vi "ajouterdonneeuser.vi"(0 "Validation":bool, 1 "Nom":string, 2 "Fichier DB":string, 3 "Prénom":string, 4 "Code du poste":dbl) -> ()   [LabVIEW 2024]
uses:
  <vilib>/drjdpowell/SQLite Library/SQL Connection/Open (string).vi
  <vilib>/drjdpowell/SQLite Library/SQL Connection/Execute SQL (No results).vi
  <vilib>/drjdpowell/SQLite Library/SQL Connection/Connection.lvclass
  <vilib>/drjdpowell/SQLite Library/SQLite.lvlib
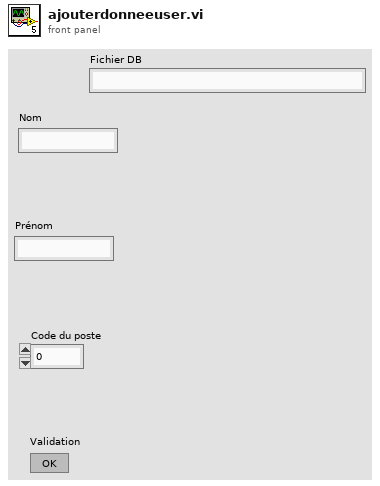
[diagram p1: front panel]
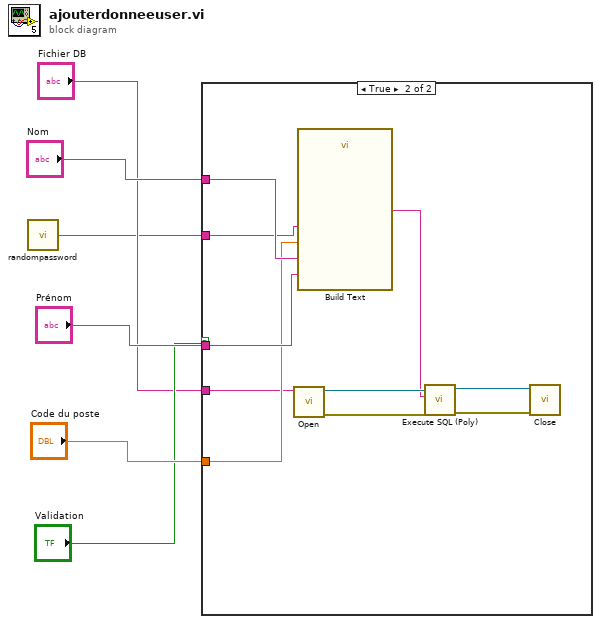
[diagram p0: block diagram]
diagram:
  n1 = call "randompassword.vi"() -> ("Password"=w1:string)
  n2 = case shown="True" "Validation" {
    tunnel: "Nom" -> [_ w11]
    tunnel: "Prénom" -> [_ w10]
    tunnel: "Code du poste" -> [_ w9]
    tunnel: "Fichier DB" -> [_ w8]
    tunnel: w1 -> [_ w7]
    frame False {
    }
    frame True {
      n3 = call-poly <vilib>:"Open.vi"("db file"=w8) -> ("error out"=w15:errorcluster, "SQLite Connection"=w16:refnum<class "Connection.lvclass">)  [unwired: 9 in]
      n4 = call "Build Text"("prenom"=w10, "password"=w7, "poste"=w9, "nom"=w11) -> ("Result"=w14:string)  [unwired: 10 in, 1 out]
      n5 = call-poly <vilib>:"Execute SQL (Poly).vi"("error in (no error)"=w15, "SQL"=w14, "SQLite Connection in"=w16) -> ("error out"=w13:errorcluster, "SQLite Connection"=w12:refnum<class "Connection.lvclass">)  [unwired: 7 in]
      n6 = call-dynamic "Close.vi"("error in (no error)"=w13, "SQLite Connection in"=w12) -> ()  [unwired: 9 in, 1 out]
    }
  }
